vi "Run.vi"(8 "error in (no error)":errorcluster caption="entrée d'erreur (pas d'erreur)", 11 "Checkerboard.lvclass":refnum<class "Checkerboard.lvclass">) -> (0 "error out":errorcluster caption="sortie d'erreur", 2 "Data":T1, 3 "Checkerboard.lvclass":refnum<class "Checkerboard.lvclass">)   [LabVIEW 2020, in "Checkerboard.lvclass"]
doc: "Returns : \n\nX : array of shape shape\n The generated array.\n\nrows : array of shape (n_clusters, X.shape[0],)\n The indicators for cluster membership of each row.\n\ncols : array of shape (n_clusters, X.shape[1],)\n The indicators for cluster membership of each column."
uses:
  Checkerboard.lvclass
  Checkerboard.lvclass/Checkerboard.ctl
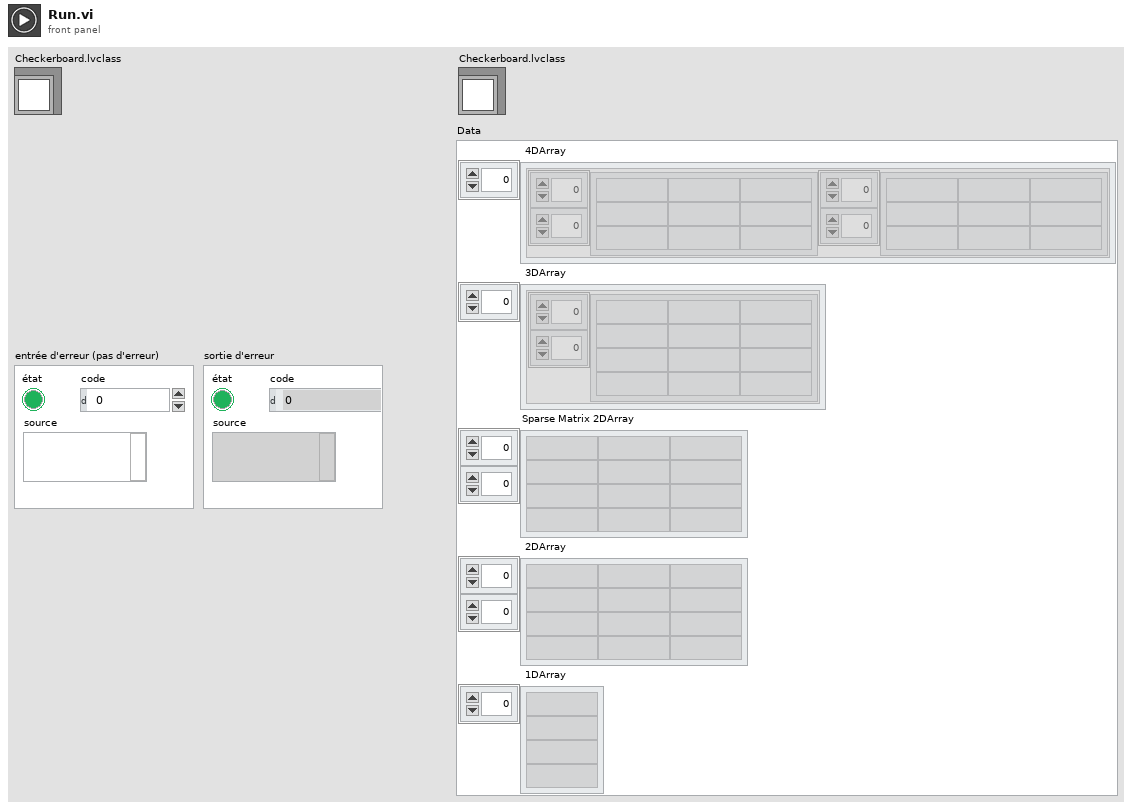
[diagram p1: front panel]
types:
  T1 = cluster{" 4DArray":cluster{"1":string[][], "2":string[][]}[], " 3DArray":cluster{"Tableau":string[][]}[], "Sparse Matrix 2DArray":string[][], " 2DArray":string[][], " 1DArray":string[]}
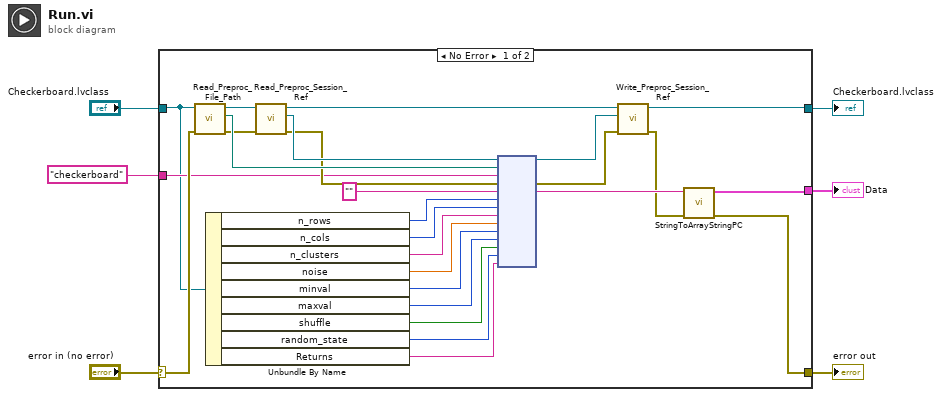
[diagram p0: block diagram]
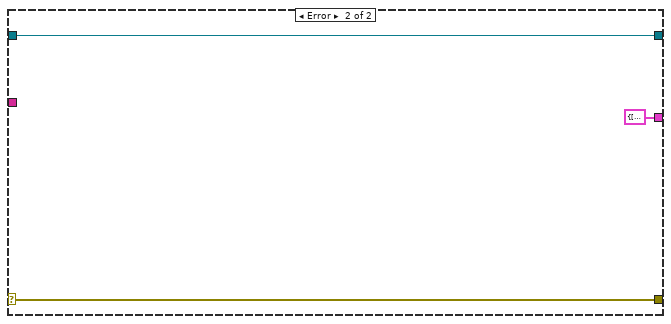
[diagram p2: hidden frame]
diagram:
  n1 = case shown="No Error" "error in (no error)" {
    selector: "error in (no error)" -> [w15 w35]
    tunnel: [w8 w35] -> w5
    tunnel: [w11 w34] -> w3
    tunnel: "Checkerboard.lvclass" -> [w13 w34]
    tunnel: "checkerboard" -> [w14 _]
    tunnel: [w7 T1 {" 4DArray"=[], " 3DArray"=[], "Sparse Matrix 2DArray"=[], " 2DArray"=[], " 1DArray"=[]} ("Data")] -> w1
    frame No Error {
      n2 = call-dynamic "Read_Preproc_File_Path.vi"("error in (no error)"=w15, "Python in"=w13) -> ("error out"=w27:errorcluster, "File_Path"=w30:path, "Python out"=w32:refnum<class "Checkerboard.lvclass">)  [unwired: 7 in]
      n3 = Unbundle By Name(w13) -> ("n_rows"=w23:u32, "n_cols"=w22:u32, "n_clusters"=w21:string, "noise"=w20:dbl, "minval"=w19:i32, "maxval"=w18:i32, "shuffle"=w17:bool, "random_state"=w16:i32, "Returns"=w12:string)
      n4 = call-dynamic "Read_Preproc_Session_Ref.vi"("error in (no error)"=w27, "Python in"=w32) -> ("error out"=w28:errorcluster, "Session_ref"=w29:refnum<k35>, "Python out"=w31:refnum<class "Checkerboard.lvclass">)  [unwired: 7 in]
      n5 = node(w29, w30, w14, w28, "", w23, w22, w21, w20, w19, w18, w17, w16, w12) -> (w24:refnum<k35>, w26:errorcluster, w10:string)  [unwired: 9 in, 2 out]
      n6 = call-dynamic "Write_Preproc_Session_Ref.vi"("error in (no error)"=w26, "Session_ref"=w24, "Python in"=w31) -> ("error out"=w9:errorcluster, "Python out"=w11:refnum<class "Checkerboard.lvclass">)  [unwired: 7 in]
      n7 = call "StringToArrayStringPC.vi"("sortie d'erreur"=w9, "Return value"=w10) -> ("sortie d'erreur"=w8:errorcluster, "Data"=w7:T1)  [unwired: 8 in]
    }
    frame Error {
    }
  }
  "error out" <- w5
  "Checkerboard.lvclass" <- w3
  "Data" <- w1
